vi "RTM - Add Channels Updated.vi"(8 "error in (no error)":errorcluster, 11 "Node Ptr":u64 format="%.0x") -> (0 "error out":errorcluster)   [LabVIEW 2016, in "UDP-Custom-Device System Explorer.lvlib"]
uses:
  UDP-Custom-Device System Explorer.lvlib
  <vilib>/NI Veristand/Custom Device API/Custom Device Item Ref.ctl
  <vilib>/NI Veristand/Custom Device API/Custom Device Channel Type.ctl
  Shared/Types/Shared - Channel Data Type.ctl
  <vilib>/NI VeriStand/Custom Device API/Custom Device API.lvlib
  <vilib>/NI VeriStand/Custom Device Tools/Custom Device Utility Library/Custom Device Utility Library.lvlib
  Property Accessors/Tx Packet Accessors.lvlib
  Shared/UDP-Custom-Device Shared.lvlib
  Property Accessors/Shared Packet Accessors.lvlib
panel:
  in  "Remove":bool
  in  "Selected Channels":i32[](listbox)
  in  "Add":bool
  in  "Available Channels":string[](tree)
  in  "OK":bool
  in  "Cancel":bool
  in  "Initial Selection":T1[](array[typedef]) format="%.0x"
  in  "Tag":string
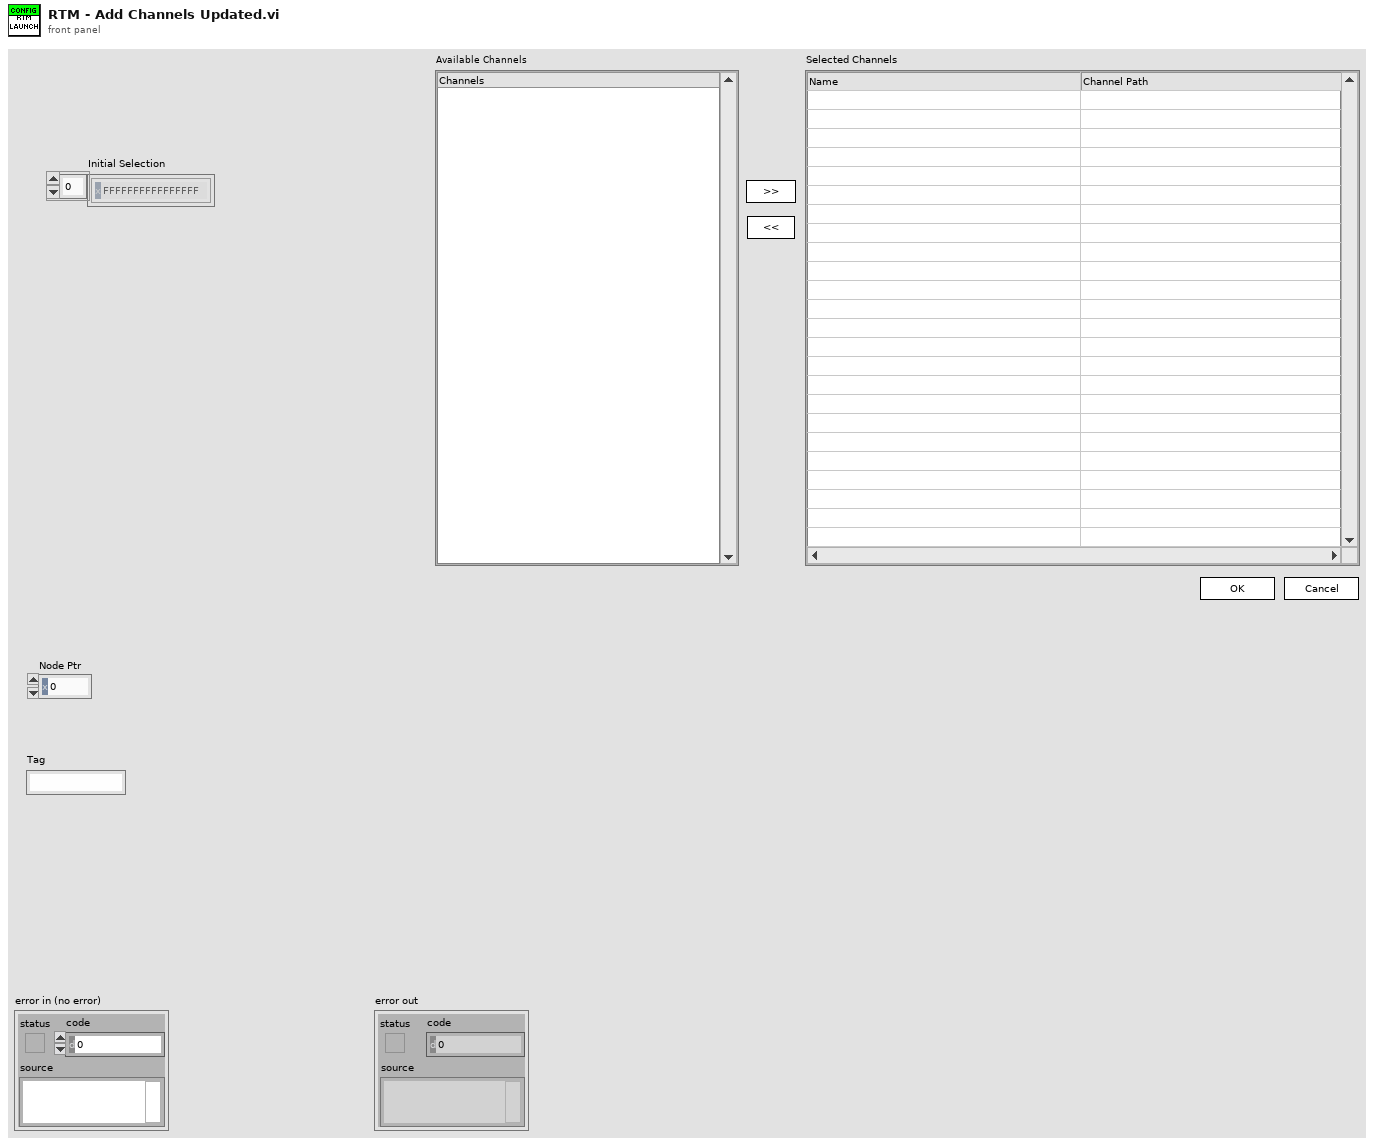
[diagram p1: front panel]
types:
  T1 = typedef "Custom Device API.lvlib/Custom Device Item Ref.ctl" = u64
  T2 = cluster{"Allow Section Selection (F)":bool, "Allow Multiple Selection (F)":bool}
  T3 = cluster{"Available Channels Label":string, "Selected Channels Label":string, "Mode":enum16{"Tx", "Rx"}}
  T4 = enum8{"Enabled", "Disabled", "Disabled and Grayed Out"}
  T5 = typedef "UDP-Custom-Device Shared.lvlib/Shared - Channel Data Type.ctl" = enum16{"Boolean", "Single", "Double", "I8", "I16", "I32", "I64", "U8", "U16", "U32", "U64"}
  T6 = typedef "Custom Device API.lvlib/Custom Device Channel Type.ctl" = enum16{"Input", "Output"}
  T7 = typedef "LVRowAndColumnUnsignedTypeDef.ctl" = cluster{"Row":u32, "Column":u32}
  T8 = typedef "Custom Device API.lvlib/Custom Device Item Info.ctl" = cluster{"Name":string, "Is Channel":bool, "GUID":string, "Is Waveform":bool}
  T9 = typedef "Custom Device API.lvlib/Custom Device Channel.ctl" = cluster{"Type":T6, "Units":string, "Default Value":dbl, "Faultable":bool, "Scalable":bool}
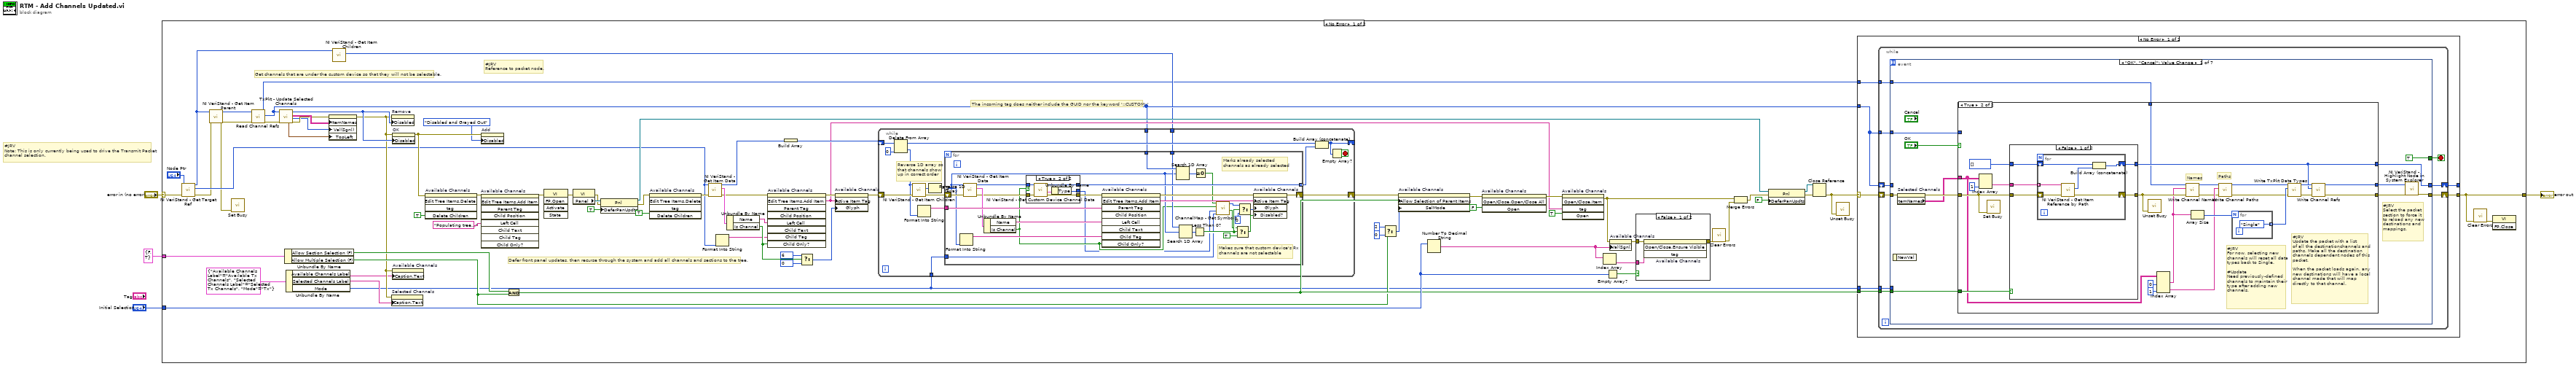
[diagram p0: block diagram]
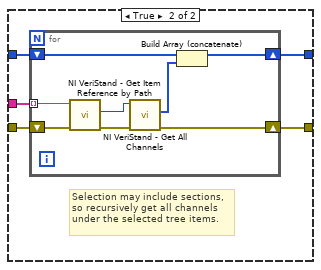
[diagram p4: hidden frame]
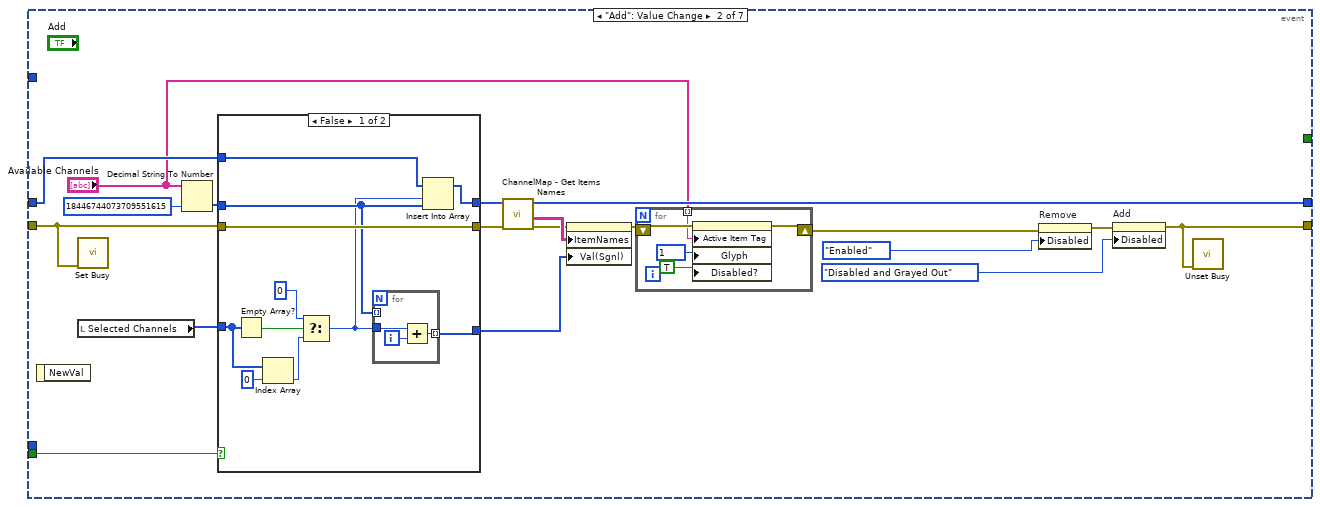
[diagram p5: hidden frame]
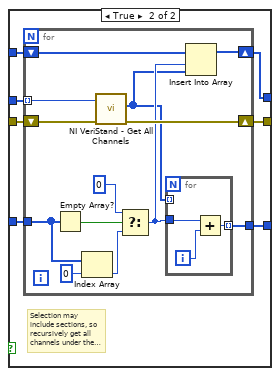
[diagram p6: hidden frame]
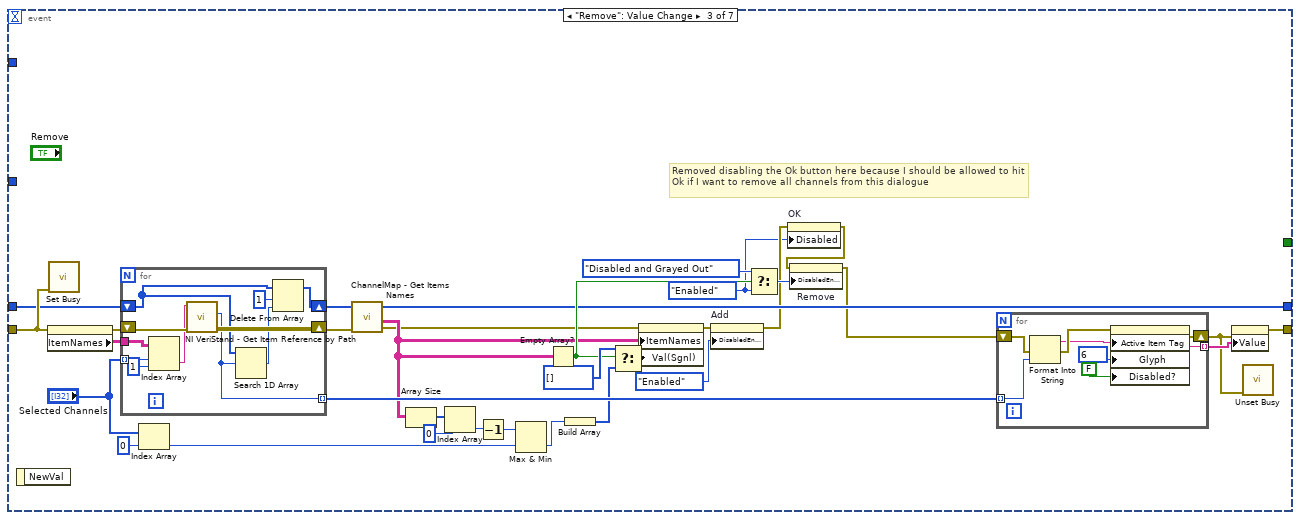
[diagram p7: hidden frame]
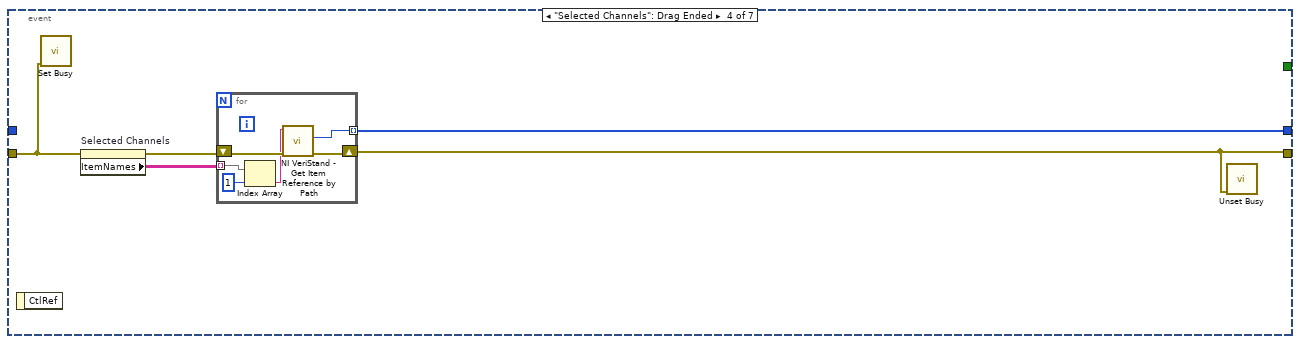
[diagram p8: hidden frame]
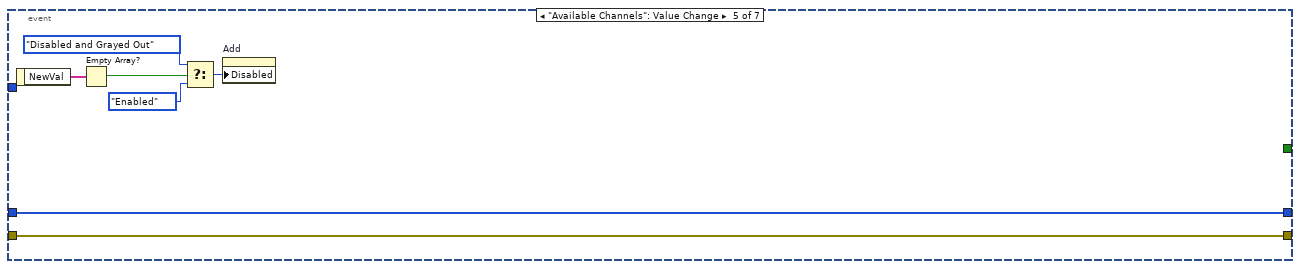
[diagram p9: hidden frame]
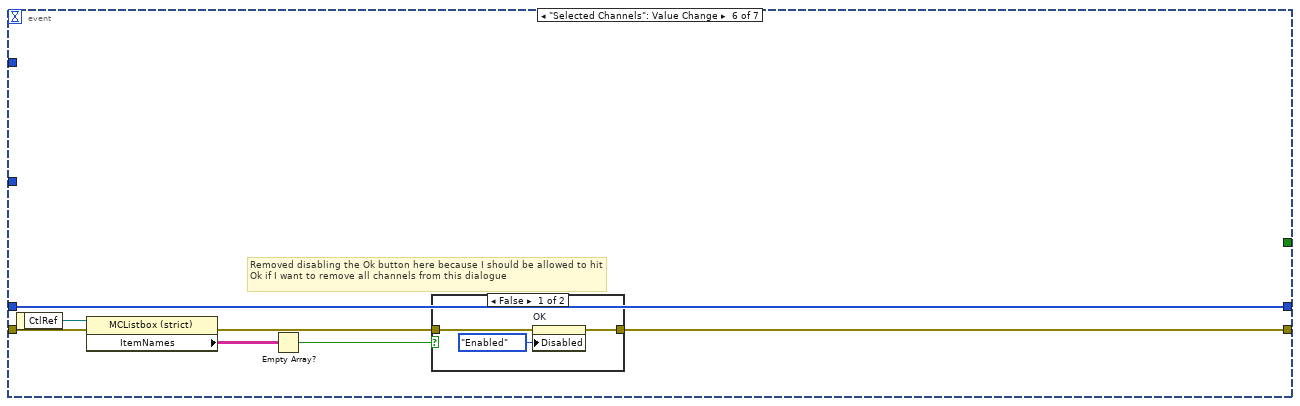
[diagram p10: hidden frame]
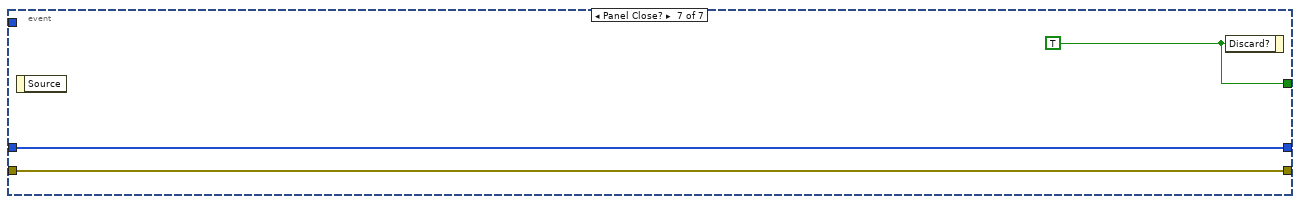
[diagram p12: hidden frame]
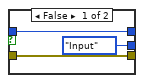
[diagram p14: hidden frame]
diagram:
  # "#JRV\nNote: This is only currently being used to drive the Transmit Packet\nchannel selection."
  # "The incoming tag does neither include the GUID nor the keyword '::CUSTOM::'"
  n1 = case shown="No Error" "error in (no error)" {
    selector: "error in (no error)" -> [w15 w361]
    tunnel: "Initial Selection" -> [w45 _]
    tunnel: [w63 w361] -> w1
    tunnel: T2 {"Allow Section Selection (F)"=FALSE, "Allow Multiple Selection (F)"=TRUE} ("Cluster") -> [w30 _]
    frame No Error {
      # "#JRV\nReference to packet node."
      # "Get channels that are under the custom device so that they will not be selectable."
      # "Defer front panel updates, then recurse through the system and add all channels and sections to the tree."
      n2 = call <vilib>:"NI VeriStand - Get Target Ref.vi"("error in"=w15, "Item Ref in"="Node Ptr") -> ("error out"=w12:errorcluster, "Target Ref"=w13:T1, "Item Ref out"=w9:T1)  [unwired: 6 in, 1 out]
      n3 = call <vilib>:"NI VeriStand - Get Item Parent.vi"("error in (no error)"=w12, "Item Ref in"=w9) -> ("error out"=w6:errorcluster, "Item Ref out"=w8:T1)  [unwired: 6 in, 2 out]
      n4 = call <vilib>:"Set Busy.vi"("error in (no error)"=w6) -> ()  [unwired: 3 in, 8 out]
      n5 = call "Read Channel Refs.vi"("error in (no error)"=w6, "Node Ptr"=w8) -> ("error out"=w16:errorcluster, "Dependent Node Refs"=w17:T1[], "Node Ptr out"=w7:T1)  [unwired: 7 in]
      n6 = call "TxPkt - Update Selected Channels.vi"("error in (no error)"=w16, "Dependent Node Refs"=w17) -> ("error out"=w26:errorcluster, "Val(Sgnl)"=w22:i32[], "Selected Channels"=w27:string[][], "Disabled Behavior"=w23:u8, "Top Left Visible Cell"=w11:T7)  [unwired: 5 in]
      n7 = Unbundle By Name(w30) -> ("Allow Section Selection (F)"=w29:bool, "Allow Multiple Selection (F)"=w28:bool)
      n8 = Unbundle By Name(T3 {"Available Channels Label"="Available Tx Channels", "Selected Channels Label"="Selected Tx Channels", "Mode"=enum."Tx"} ("Parameter")) -> ("Available Channels Label"=w20:string, "Selected Channels Label"=w19:string, "Mode"=w18:enum16{"Tx", "Rx"})
      n9 = property on="Selected Channels" class="MCListbox (strict)"(error in=w26, "ItemNames"=w27, "Val(Sgnl)"=w22, "TopLeft"=w11) -> (error out=w21:errorcluster)  [unwired: 1 in, 1 out]
      n10 = call <vilib>:"NI VeriStand - Get Item Children.vi"("Item Ref in"=w9) -> ("Child Refs"=w10:T1[])  [unwired: 7 in, 3 out]
      n11 = property on="Remove" class="Bool"(error in=w21, "Disabled"=w23) -> ()  [unwired: 1 in, 2 out]
      n12 = property on="Selected Channels" class="MCListbox (strict)"(error in=w21, "Caption.Text"=w19) -> ()  [unwired: 1 in, 2 out]
      n13 = property on="OK" class="Bool"(error in=w21, "Disabled"=w23) -> (error out=w25:errorcluster)  [unwired: 1 in, 1 out]
      n14 = property on="Available Channels" class="Tree (strict)"(error in=w21, "Caption.Text"=w20) -> ()  [unwired: 1 in, 2 out]
      n15 = invoke on="Available Channels" class="Tree (strict)" method="Edit Tree Items.Delete"(error in=w25, "Delete Children"=TRUE ("Delete Children?")) -> (error out=w79:errorcluster)  [unwired: 3 in, 4 out]
      n16 = invoke on="Available Channels" class="Tree (strict)" method="Edit Tree Items.Add Item"(error in=w79, "Left Cell"="Populating tree..." ("Tag")) -> (error out=w76:errorcluster)  [unwired: 7 in, 8 out]
      n17 = property on="Add" class="Bool"(error in=w25, "Disabled"=T4."Disabled and Grayed Out") -> ()  [unwired: 1 in, 2 out]
      n18 = Compound Arithmetic op=AND(w29, w28) -> (w32:bool)
      n19 = invoke class="VI" method="FP.Open"(error in=w76) -> (error out=w74:errorcluster)  [unwired: 4 in, 4 out]
      n20 = property class="VI"(error in=w74) -> (error out=w72:errorcluster, "Panel"=w73:refnum<vi>)  [unwired: 1 in, 1 out]
      n21 = property class="Pnl"(reference=w73, error in=w72, "DeferPanUpdts"=TRUE ("Defer Panel Updates")) -> (reference out=w66:refnum<vi>, error out=w70:errorcluster)
      n22 = invoke on="Available Channels" class="Tree (strict)" method="Edit Tree Items.Delete"(error in=w70, "Delete Children"=TRUE ("Delete Children?")) -> (error out=w50:errorcluster)  [unwired: 3 in, 4 out]
      n23 = call <vilib>:"NI VeriStand - Get Item Data.vi"("error in (no error)"=w50, "Item Ref in"=w13) -> ("error out"=w53:errorcluster, "Item Info"=w55:T8, "Item Ref out"=w51:T1)  [unwired: 7 out]
      n24 = Format Into String(w13) -> (resulting string=w54:string)  [unwired: 3 in, 1 out]
      n25 = Unbundle By Name(w55) -> ("Name"=w56:string, "Is Channel"=w60:bool)
      n26 = invoke on="Available Channels" class="Tree (strict)" method="Edit Tree Items.Add Item"(error in=w53, "Left Cell"=w56, "Child Tag"=w54, "Child Only?"=w60) -> (error out=w57:errorcluster, "Edit Tree Items:Add Item"=w36:string)  [unwired: 5 in, 7 out]
      n27 = Build Array(w51) -> (w69:T1[])
      n28 = Select(t=6, s=w60, f=0) -> (s? t:f=w61:i32)
      n29 = property on="Available Channels" class="Tree (strict)"(error in=w57, "Active Item Tag"=w36, "Glyph"=w61) -> (error out=w52:errorcluster)  [unwired: 1 in, 1 out]
      n30 = while {
        shift-right: [w314] -> w68
        shift-left: w52 -> [w320]
        shift-right: [w319] -> _
        shift-left: w69 -> [w323]
        tunnel: w17 -> [w311]
        tunnel: w18 -> [w310]
        tunnel: w10 -> [w309]
        stop <- w318 stop-if-true
        # "Reverse 1D array so that channels show up in correct order"
        n31 = Delete From Array(array=w323, index=0) -> (deleted portion=w313:T1, array with subset deleted=w321:T1[])  [unwired: 1 in]
        n32 = call <vilib>:"NI VeriStand - Get Item Children.vi"("error in (no error)"=w320, "Item Ref in"=w313) -> ("error out"=w317:errorcluster, "Child Refs"=w316:T1[])  [unwired: 8 out]
        n33 = Format Into String(w313) -> (resulting string=w312:string)  [unwired: 3 in, 1 out]
        n34 = Reverse 1D Array(array=w316) -> (reversed array=w308:T1[])
        n35 = for {
          shift-right: [w345] -> w314
          shift-left: w317 -> [w350]
          tunnel: w308 -> [w337] mode=indexing
          tunnel: [w342] -> w315 mode=indexing
          tunnel: w312 -> [w351]
          tunnel: w311 -> [w344]
          tunnel: w310 -> [w326]
          tunnel: w309 -> [w338]
          # "Marks already selected channels as already selected"
          # "Makes sure that custom device's Rx channels are not selectable"
          n36 = Format Into String(w337) -> (resulting string=w349:string)  [unwired: 3 in, 1 out]
          n37 = call <vilib>:"NI VeriStand - Get Item Data.vi"("error in (no error)"=w350, "Item Ref in"=w337) -> ("error out"=w341:errorcluster, "Item Info"=w348:T8, "Item Ref out"=w343:T1)  [unwired: 7 out]
          n38 = Unbundle By Name(w348) -> ("Name"=w339:string, "Is Channel"=w328:bool)
          n39 = case shown="True" w328 {
            tunnel: w343 -> [w354 w360]
            tunnel: [w354 w359] -> w342
            tunnel: w341 -> [w353 w358]
            tunnel: [w353 w357] -> w340
            tunnel: [Custom_Device_Channel_Type."Input" ("Type") w355] -> w327
            frame False {
            }
            frame True {
              n40 = call <vilib>:"NI VeriStand - Get Custom Device Channel Data.vi"("error in (no error)"=w358, "Channel Ref in"=w360) -> ("error out"=w357:errorcluster, "Channel"=w356:T9, "Channel Ref out"=w359:T1)  [unwired: 4 in, 3 out]
              n41 = Unbundle By Name(w356) -> ("Type"=w355:T6)
            }
          }
          n42 = invoke on="Available Channels" class="Tree (strict)" method="Edit Tree Items.Add Item"(error in=w340, "Parent Tag"=w351, "Left Cell"=w339, "Child Tag"=w349, "Child Only?"=w328) -> (error out=w347:errorcluster, "Edit Tree Items:Add Item"=w346:string)  [unwired: 4 in, 7 out]
          n43 = Search 1D Array(1D array=w344, element=w337) -> (index of element=w330:i32)  [unwired: 1 in]
          n44 = Search 1D Array(1D array=w338, element=w337) -> (index of element=w336:i32)  [unwired: 1 in]
          n45 = Less Than 0?(x=w336) -> (x < 0?=w332:bool)
          n46 = Greater Or Equal To 0?(x=w330) -> (x >= 0?=w329:bool)
          n47 = call "ChannelMap - Get Symbols.vi"("Mode"=w326, "Channel Type"=w327, "Is Channel?"=w328, "Is Selected?"=w329) -> ("Disabled?"=w324:bool, "Symbole"=w325:i32)  [unwired: 6 in]
          n48 = Select(t=w324, s=w332, f=TRUE) -> (s? t:f=w335:bool)
          n49 = Select(t=w325, s=w332, f=0) -> (s? t:f=w333:i32)
          n50 = property on="Available Channels" class="Tree (strict)"(error in=w347, "Active Item Tag"=w346, "Glyph"=w333, "Disabled?"=w335) -> (error out=w345:errorcluster)  [unwired: 1 in, 1 out]
        }
        n51 = Build Array (concatenate)(w321, w315) -> (w319:T1[])
        n52 = Empty Array?(array=w319) -> (empty?=w318:bool)
      }
      n53 = Select(t=2 ("Selection Mode"), s=w28, f=0 ("Selection Mode")) -> (s? t:f=w33:i32)
      n54 = property on="Available Channels" class="Tree (strict)"(error in=w68, "Allow Selection of Parent Items"=w32, "SelMode"=w33) -> (error out=w41:errorcluster)  [unwired: 1 in, 1 out]
      n55 = Number To Decimal String(number=w45) -> (decimal integer string=w43:string[])  [unwired: 1 out]
      n56 = invoke on="Available Channels" class="Tree (strict)" method="Open/Close.Open/Close All"(error in=w41, "Open"=FALSE ("Open?")) -> (error out=w39:errorcluster)  [unwired: 2 in, 3 out]
      n57 = invoke on="Available Channels" class="Tree (strict)" method="Open/Close.Item"(error in=w39, "tag"=w36, "Open"=TRUE ("Open?")) -> (error out=w37:errorcluster)  [unwired: 2 in, 4 out]
      n58 = Index Array(array=w43) -> (element=w42:string)  [unwired: 1 in]
      n59 = Empty Array?(array=w45) -> (empty?=w44:bool)
      n60 = property on="Available Channels" class="Tree (strict)"(error in=w37, "Val(Sgnl)"=w43) -> (error out=w47:errorcluster)  [unwired: 1 in, 1 out]
      n61 = case shown="False" w44 {
        tunnel: w47 -> [w82 w83]
        tunnel: [w81 w83] -> w46
        tunnel: w42 -> [w80 _]
        frame False {
          n62 = invoke on="Available Channels" class="Tree (strict)" method="Open/Close.Ensure Visible"(error in=w82, "tag"=w80) -> (error out=w81:errorcluster)  [unwired: 2 in, 3 out]
        }
        frame True {
        }
      }
      n63 = call <vilib>:"Clear Errors.vi"("error in (no error)"=w46) -> ("error out"=w49:errorcluster)  [unwired: 1 in, 5 out]
      n64 = Merge Errors(w37, w49) -> (w48:errorcluster)
      n65 = property class="Pnl"(reference=w66, error in=w48, "DeferPanUpdts"=FALSE ("Defer Panel Updates")) -> (reference out=w64:refnum<vi>, error out=w65:errorcluster)
      n66 = Close Reference(reference=w64, error in (no error)=w65) -> (error out=w31:errorcluster)
      n67 = call <vilib>:"Unset Busy.vi"("error in (no error)"=w31) -> ()  [unwired: 1 in, 10 out]
      n68 = case shown="No Error" w31 {
        selector: w31 -> [w90 w307]
        tunnel: [w89 w307] -> w63
        tunnel: [w88 w306] -> _
        tunnel: w32 -> [w87 _]
        tunnel: w17 -> [w86 w306]
        tunnel: w18 -> [w85 _]
        tunnel: w7 -> [w84 _]
        frame No Error {
          n69 = while {
            shift-right: [w98] -> w89
            shift-left: w90 -> [w99]
            tunnel: w87 -> [w96]
            shift-right: [w93] -> w88
            shift-left: w86 -> [w95]
            tunnel: w86 -> [w94]
            tunnel: w85 -> [w92]
            tunnel: w84 -> [w91]
            stop <- w97 stop-if-true
            n70 = event shown="[0] \"OK\", \"Cancel\": Value Change" {
              selector: _ -> [_ _ _ _ _ _ _]
              dyn-events: _ -> [_ _ _ _ _ _ _]
              timeout: _ -> [_ _ _ _ _ _ _]
              tunnel: w99 -> [w108 w179 w255 w278 w291 w296 w305]
              tunnel: [w104 w163 w228 w275 w291 w293 w305] -> w98
              tunnel: [TRUE ("Discard?") _ _ _ _ _ w304] -> w97
              tunnel: [w100 w175 w234 w274 w288 w298 w303] -> w93
              tunnel: w96 -> [w110 w178 _ _ _ _ _]
              tunnel: w95 -> [_ w177 w252 _ w288 w298 w303]
              tunnel: w94 -> [w106 _ _ _ _ _ _]
              tunnel: w92 -> [_ _ _ _ _ _ _]
              tunnel: w91 -> [w103 _ _ _ _ _ _]
              event "OK", "Cancel": Value Change {
                # "#JRV\nSelect the packet\nsection to force it\nto reload any new\ndestinations and\nmappings."
                n71 = event-data() -> ()  [unwired: 2 out]
                n72 = property on="Selected Channels" class="MCListbox (strict)"(error in=w108) -> (error out=w107:errorcluster, "ItemNames"=w105:string[][])  [unwired: 1 in, 1 out]
                n73 = case shown="True" "OK" {
                  tunnel: w105 -> [_ w130]
                  tunnel: w110 -> [_ w137]
                  tunnel: w107 -> [w114 w135]
                  tunnel: [w113 w118] -> w100
                  tunnel: [w114 w117] -> w101
                  tunnel: w106 -> [w113 _]
                  tunnel: w103 -> [w112 w115]
                  tunnel: [w112 w116] -> w102
                  frame False {
                  }
                  frame True {
                    # "#JRV\nFor now, selecting new\nchannels will reset all data\ntypes back to Single.\n\n#Update\nNeed previously-defined\nchannels to maintain their\ntype after adding new\nchannels."
                    # "Paths"
                    # "Names"
                    # "#JRV\nUpdate the packet with a list\nof all the destinationchannels and\npaths. Make all the destination\nchannels dependent nodes of this\npacket.\n\nWhen the packet loads again, any\nnew destinations will have a local\nchannel made that will map\ndirectly to that channel."
                    n74 = Index Array(array=w130, index (col)=1 ("disabled index (col)")) -> (element=w133:string[])  [unwired: 1 in]
                    n75 = call <vilib>:"Set Busy.vi"("error in (no error)"=w135) -> ()  [unwired: 3 in, 8 out]
                    n76 = case shown="False" w137 {
                      tunnel: w135 -> [w143 w154]
                      tunnel: [w139 w152] -> w118
                      tunnel: [w142 w151] -> w127
                      tunnel: T1[] [] ("Channel Refs") -> [w140 w153]
                      tunnel: w133 -> [w141 w150]
                      frame False {
                        n77 = for {
                          tunnel: w141 -> [w147] mode=indexing
                          shift-right: [w144] -> w139
                          shift-left: w140 -> [w145]
                          shift-right: [w148] -> w142
                          shift-left: w143 -> [w149]
                          n78 = call <vilib>:"NI VeriStand - Get Item Reference by Path.vi"("error in (no error)"=w149, "Item Path in"=w147) -> ("error out"=w148:errorcluster, "Item Ref"=w146:T1)  [unwired: 6 in, 2 out]
                          n79 = Build Array (concatenate)(w145, w146) -> (w144:T1[])
                        }
                      }
                      frame True {
                        # "Selection may include sections,\nso recursively get all channels\nunder the selected tree items."
                        n80 = for {
                          shift-right: [w160] -> w152
                          shift-left: w153 -> [w161]
                          shift-right: [w162] -> w151
                          shift-left: w154 -> [w157]
                          tunnel: w150 -> [w158] mode=indexing
                          n81 = call <vilib>:"NI VeriStand - Get Item Reference by Path.vi"("error in (no error)"=w157, "Item Path in"=w158) -> ("error out"=w156:errorcluster, "Item Ref"=w155:T1)  [unwired: 6 in, 2 out]
                          n82 = call <vilib>:"NI VeriStand - Get All Channels.vi"("error in"=w156, "Section Ref in"=w155) -> ("error out"=w162:errorcluster, "Channel Refs"=w159:T1[])  [unwired: 8 out]
                          n83 = Build Array (concatenate)(w161, w159) -> (w160:T1[])
                        }
                      }
                    }
                    n84 = call <vilib>:"Unset Busy.vi"("error in (no error)"=w127) -> ()  [unwired: 1 in, 10 out]
                    n85 = Index Array(array=w130, index (col) #1=0 ("disabled index (col)"), index (col) #2=1 ("index (col)")) -> (element #1=w126:string[], element #2=w124:string[])  [unwired: 2 in]
                    n86 = call "Write Channel Names.vi"("error in (no error)"=w127, "Channel Names"=w126, "Node Ptr"=w115) -> ("error out"=w123:errorcluster, "Node Ptr out"=w125:T1)  [unwired: 7 in]
                    n87 = Array Size(array=w126) -> (size(s)=w129:i32)
                    n88 = call "Write Channel Paths.vi"("error in (no error)"=w123, "Channel Paths"=w124, "Node Ptr"=w125) -> ("error out"=w122:errorcluster, "Node Ptr out"=w121:T1)  [unwired: 7 in]
                    n89 = for {
                      N: w129 -> [_]
                      tunnel: [Shared_-_Channel_Data_Type."Single" ("Data Type")] -> w128 mode=indexing
                    }
                    n90 = call "Write TxPkt Data Types.vi"("error in (no error)"=w122, "Data Types"=w128, "Node Ptr"=w121) -> ("error out"=w119:errorcluster, "Node Ptr out"=w120:T1)  [unwired: 7 in]
                    n91 = call "Write Channel Refs.vi"("error in (no error)"=w119, "Dependent Node Refs"=w118, "Node Ptr"=w120) -> ("error out"=w117:errorcluster, "Node Ptr out"=w116:T1)  [unwired: 7 in]
                  }
                }
                n92 = call <vilib>:"NI VeriStand - Highlight Node in System Explorer.vi"("error in (no error)"=w101, "Item Ref in"=w102) -> ("error out"=w104:errorcluster)  [unwired: 8 in, 1 out]
              }
              event "Add": Value Change {
                n93 = event-data() -> ()  [unwired: 2 out]
                n94 = call <vilib>:"Set Busy.vi"("error in (no error)"=w179) -> ()  [unwired: 3 in, 8 out]
                n95 = local read "Selected Channels"() -> (w167:i32[])
                n96 = Decimal String To Number(string="Available Channels", default (0L)=T1 18446744073709551615 ("Device Item Ref")) -> (number=w181:u64[])  [unwired: 2 out]
                n97 = case shown="False" w178 {
                  tunnel: w179 -> [w197 w207]
                  tunnel: [w194 w206] -> w176
                  tunnel: w181 -> [w189 w205]
                  tunnel: [w197 w204] -> w174
                  tunnel: w177 -> [w195 w203]
                  tunnel: w167 -> [w193 w202]
                  tunnel: [w187 w201] -> w166
                  frame False {
                    n98 = Empty Array?(array=w193) -> (empty?=w196:bool)
                    n99 = Index Array(array=w193, index=0) -> (element=w191:i32)
                    n100 = Select(t=0, s=w196, f=w191) -> (s? t:f=w188:i32)
                    n101 = for {
                      tunnel: w189 -> [_] mode=indexing
                      tunnel: w188 -> [w200]
                      tunnel: [w198] -> w187 mode=indexing
                      i -> [w199]
                      n102 = Add(x=w200, y=w199) -> (x+y=w198:i32)
                    }
                    n103 = Insert Into Array(array=w195, index=w188, new element=w189) -> (w194:T1[])
                  }
                  frame True {
                    # "Selection may include sections, so recursively get all channels under the selected tree items."
                    n104 = for {
                      shift-right: [w212] -> w206
                      shift-left: w203 -> [w211]
                      shift-right: [w219] -> w204
                      shift-left: w207 -> [w220]
                      tunnel: w205 -> [w218] mode=indexing
                      tunnel: w202 -> [w213]
                      tunnel: [w210] -> w201
                      n105 = Empty Array?(array=w213) -> (empty?=w214:bool)
                      n106 = Index Array(array=w213, index=0) -> (element=w216:i32)
                      n107 = call <vilib>:"NI VeriStand - Get All Channels.vi"("error in"=w220, "Section Ref in"=w218) -> ("error out"=w219:errorcluster, "Channel Refs"=w208:T1[])  [unwired: 8 out]
                      n108 = Select(t=0, s=w214, f=w216) -> (s? t:f=w209:i32)
                      n109 = for {
                        tunnel: w209 -> [w223]
                        tunnel: [w221] -> w210 mode=indexing
                        tunnel: w208 -> [_] mode=indexing
                        i -> [w222]
                        n110 = Add(x=w223, y=w222) -> (x+y=w221:i32)
                      }
                      n111 = Insert Into Array(array=w211, index=w209, new element=w208) -> (w212:T1[])
                    }
                  }
                }
                n112 = call "ChannelMap - Get Items Names.vi"("error IO 2"=w174, "TCP Channel Refs In"=w176) -> ("error IO"=w169:errorcluster, "Items Names"=w170:string[][], "TCP Channel Refs Out"=w175:T1[])  [unwired: 7 in]
                n113 = property on="Selected Channels" class="MCListbox (strict)"(error in=w169, "ItemNames"=w170, "Val(Sgnl)"=w166) -> (error out=w173:errorcluster)  [unwired: 1 in, 1 out]
                n114 = for {
                  shift-right: [w185] -> w165
                  shift-left: w173 -> [w186]
                  tunnel: "Available Channels" -> [w183] mode=indexing
                  n115 = property on="Available Channels" class="Tree (strict)"(error in=w186, "Active Item Tag"=w183, "Glyph"=1, "Disabled?"=TRUE ("Active Item:Disabled?")) -> (error out=w185:errorcluster)  [unwired: 1 in, 1 out]
                }
                n116 = property on="Remove" class="Bool"(error in=w165, "Disabled"=T4."Enabled") -> (error out=w164:errorcluster)  [unwired: 1 in, 1 out]
                n117 = property on="Add" class="Bool"(error in=w164, "Disabled"=T4."Disabled and Grayed Out") -> (error out=w163:errorcluster)  [unwired: 1 in, 1 out]
                n118 = call <vilib>:"Unset Busy.vi"("error in (no error)"=w163) -> ()  [unwired: 1 in, 10 out]
              }
              event "Remove": Value Change {
                w225 = T4."Enabled" ("Disabled")
                # "Removed disabling the Ok button here because I should be allowed to hit Ok if I want to remove all channels from this dialogue"
                n119 = event-data() -> ()  [unwired: 2 out]
                n120 = property on="Selected Channels" class="MCListbox (strict)"(error in=w255) -> (error out=w254:errorcluster, "ItemNames"=w253:string[][])  [unwired: 1 in, 1 out]
                n121 = call <vilib>:"Set Busy.vi"("error in (no error)"=w255) -> ()  [unwired: 3 in, 8 out]
                n122 = for {
                  tunnel: w253 -> [w264]
                  tunnel: "Selected Channels" -> [w265] mode=indexing
                  shift-right: [w263] -> w236
                  shift-left: w254 -> [w266]
                  shift-right: [w261] -> w233
                  shift-left: w252 -> [w262]
                  tunnel: [w258] -> w251 mode=indexing
                  n123 = Index Array(array=w264, index (row)=w265, index (col)=1 ("disabled index (col)")) -> (element=w256:string)
                  n124 = call <vilib>:"NI VeriStand - Get Item Reference by Path.vi"("error in (no error)"=w266, "Item Path in"=w256) -> ("error out"=w263:errorcluster, "Item Ref"=w258:T1)  [unwired: 6 in, 2 out]
                  n125 = Search 1D Array(1D array=w262, element=w258) -> (index of element=w259:i32)  [unwired: 1 in]
                  n126 = Delete From Array(array=w262, length=1, index=w259) -> (array with subset deleted=w261:T1[])  [unwired: 1 out]
                }
                n127 = Index Array(array="Selected Channels", index=0) -> (element=w239:i32)
                n128 = call "ChannelMap - Get Items Names.vi"("error IO 2"=w236, "TCP Channel Refs In"=w233) -> ("error IO"=w232:errorcluster, "Items Names"=w235:string[][], "TCP Channel Refs Out"=w234:T1[])  [unwired: 7 in]
                n129 = Array Size(array=w235) -> (size(s)=w243:i32[])
                n130 = Index Array(array=w243, index=0) -> (element=w241:i32)
                n131 = Decrement(x=w241) -> (x-1=w240:i32)
                n132 = Max & Min(x=w240, y=w239) -> (min(x,y)=w238:i32)  [unwired: 1 out]
                n133 = Empty Array?(array=w235) -> (empty?=w248:bool)
                n134 = Build Array(w238) -> (w245:i32[])
                n135 = Select(t=i32[] [] ("Selected TCP Channels"), s=w248, f=w245) -> (s? t:f=w249:i32[])
                n136 = property on="Selected Channels" class="MCListbox (strict)"(error in=w232, "ItemNames"=w235, "Val(Sgnl)"=w249) -> ()  [unwired: 1 in, 2 out]
                n137 = property on="Add" class="Bool"(error in=w232, "DisabledEnum"=T4."Enabled" ("Disabled")) -> (error out=w231:errorcluster)  [unwired: 1 in, 1 out]
                n138 = Select(t=T4."Disabled and Grayed Out" ("Disabled"), s=w248, f=w225) -> (s? t:f=w247:T4)
                n139 = property on="OK" class="Bool"(error in=w231, "Disabled"=w225) -> (error out=w230:errorcluster)  [unwired: 1 in, 1 out]
                n140 = property on="Remove" class="Bool"(error in=w230, "DisabledEnum"=w247) -> (error out=w229:errorcluster)  [unwired: 1 in, 1 out]
                n141 = for {
                  shift-right: [w271] -> w227
                  shift-left: w229 -> [w269]
                  tunnel: w251 -> [w270] mode=indexing
                  tunnel: [w267] -> w237 mode=indexing
                  n142 = Format Into String(error in=w269, w270) -> (resulting string=w267:string, error out=w268:errorcluster)  [unwired: 2 in]
                  n143 = property on="Available Channels" class="Tree (strict)"(error in=w268, "Active Item Tag"=w267, "Glyph"=6, "Disabled?"=FALSE ("Active Item:Disabled?")) -> (error out=w271:errorcluster)  [unwired: 1 in, 1 out]
                }
                n144 = property on="Available Channels" class="Tree (strict)"(error in=w227, "Value"=w237) -> (error out=w228:errorcluster)  [unwired: 1 in, 1 out]
                n145 = call <vilib>:"Unset Busy.vi"("error in (no error)"=w227) -> ()  [unwired: 1 in, 10 out]
              }
              event "Selected Channels": Drag Ended {
                n146 = event-data() -> ()  [unwired: 2 out]
                n147 = call <vilib>:"Set Busy.vi"("error in (no error)"=w278) -> ()  [unwired: 3 in, 8 out]
                n148 = property on="Selected Channels" class="MCListbox (strict)"(error in=w278) -> (error out=w277:errorcluster, "ItemNames"=w276:string[][])  [unwired: 1 in, 1 out]
                n149 = for {
                  tunnel: w276 -> [w283] mode=indexing
                  shift-right: [w282] -> w275
                  shift-left: w277 -> [w284]
                  tunnel: [w281] -> w274 mode=indexing
                  n150 = Index Array(array=w283, index=1 ("disabled index (col)")) -> (element=w280:string)
                  n151 = call <vilib>:"NI VeriStand - Get Item Reference by Path.vi"("error in (no error)"=w284, "Item Path in"=w280) -> ("error out"=w282:errorcluster, "Item Ref"=w281:T1)  [unwired: 6 in, 2 out]
                }
                n152 = call <vilib>:"Unset Busy.vi"("error in (no error)"=w275) -> ()  [unwired: 1 in, 10 out]
              }
              event "Available Channels": Value Change {
                n153 = event-data() -> ("NewVal"=w290:string[])  [unwired: 1 out]
                n154 = Empty Array?(array=w290) -> (empty?=w287:bool)
                n155 = Select(t=T4."Disabled and Grayed Out" ("Disabled"), s=w287, f=T4."Enabled" ("Disabled")) -> (s? t:f=w289:T4)
                n156 = property on="Add" class="Bool"("Disabled"=w289) -> ()  [unwired: 2 in, 2 out]
              }
              event "Selected Channels": Value Change {
                # "Removed disabling the Ok button here because I should be allowed to hit Ok if I want to remove all channels from this dialogue"
                n157 = event-data() -> ("CtlRef"=w297:refnum<vi>)  [unwired: 1 out]
                n158 = property class="MCListbox (strict)"(reference=w297, error in=w296) -> (error out=w294:errorcluster, "ItemNames"=w295:string[][])  [unwired: 1 out]
                n159 = Empty Array?(array=w295) -> (empty?=w292:bool)
                n160 = case shown="False" w292 {
                  tunnel: w294 -> [w301 w302]
                  tunnel: [w300 w302] -> w293
                  frame False {
                    n161 = property on="OK" class="Bool"(error in=w301, "Disabled"=T4."Enabled") -> (error out=w300:errorcluster)  [unwired: 1 in, 1 out]
                  }
                  frame True {
                  }
                }
              }
              event Panel Close? {
                w304 = TRUE ("Discard?")
                n162 = event-data() -> ()  [unwired: 2 out]
                n163 = event-data("Discard?"=w304) -> ()  [unwired: 1 in, 1 out]
              }
            }
          }
        }
        frame Error {
        }
      }
      n164 = call <vilib>:"Clear Errors.vi"("error in (no error)"=w63) -> ("error out"=w62:errorcluster)  [unwired: 1 in, 5 out]
      n165 = invoke class="VI" method="FP.Close"(error in=w62) -> ()  [unwired: 2 in, 3 out]
    }
    frame Error {
    }
  }
  "error out" <- w1
